vi "websocket main.vi"(8 "error in":errorcluster, 10 "upgrade data":T1, 11 "websocket handler in":refnum<class "websocket upgrade handler.lvclass">) -> (0 "error out":errorcluster)   [LabVIEW 2013, in "websocket upgrade handler.lvclass"]
uses:
  websocket upgrade handler.lvclass
  HTTP responder/http upgrade data.ctl
  HTTP server/http request.ctl
  HTTP server/http method.ctl
  HTTP headers/http header data.ctl
  websocket upgrade handler.lvclass/websocket upgrade handler.ctl
  user plugin/websocket user plugin.lvclass
  websocket core.lvlib
  HTTP server/Basic HTTP server.lvclass
  HTTP responder/http responder.lvclass
  HTTP headers/http headers.lvlib
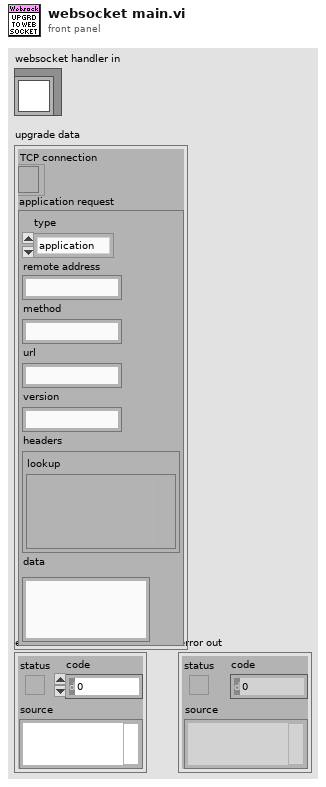
[diagram p1: front panel]
types:
  T1 = typedef "http responder.lvclass/http upgrade data.ctl" = cluster{"TCP connection":refnum<k5>, "application request":T2}
  T2 = typedef "Basic HTTP server.lvclass/http request.ctl" = cluster{"type":T3, "remote address":string, "method":string, "url":string, "version":string, "headers":T4, "data":string}
  T3 = typedef "Basic HTTP server.lvclass/http method.ctl" = enum16{"application", "error", "upgrade", "expect"}
  T4 = typedef "http headers.lvlib/http header data.ctl" = cluster{"lookup":variant}
  T5 = typedef "websocket core.lvlib/first byte header.ctl" = cluster{"fin":bool, "RSRV1":bool, "RSRV2":bool, "RSRV3":bool, "opcode":u8}
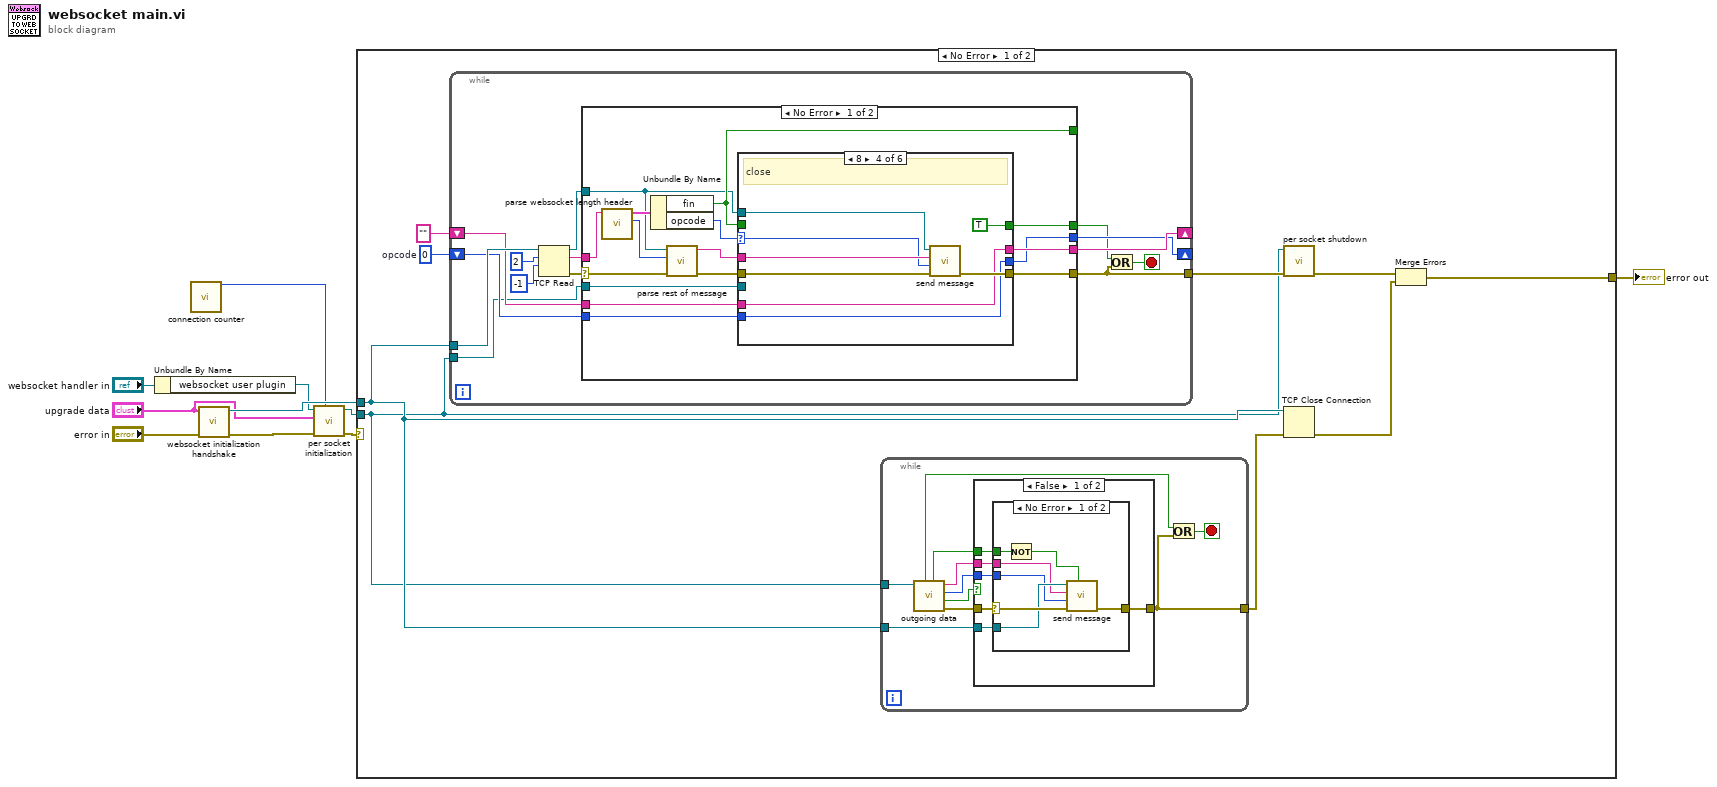
[diagram p0: block diagram]
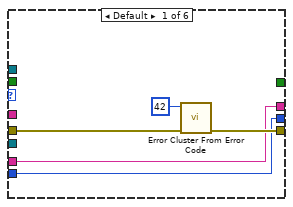
[diagram p4: hidden frame]
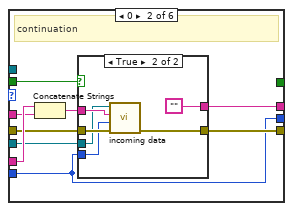
[diagram p5: hidden frame]
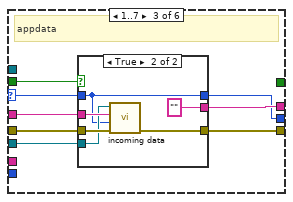
[diagram p7: hidden frame]
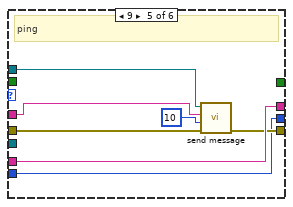
[diagram p9: hidden frame]
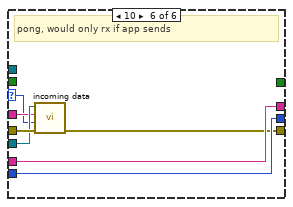
[diagram p10: hidden frame]
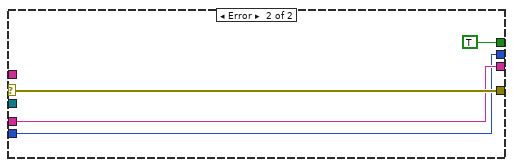
[diagram p11: hidden frame]
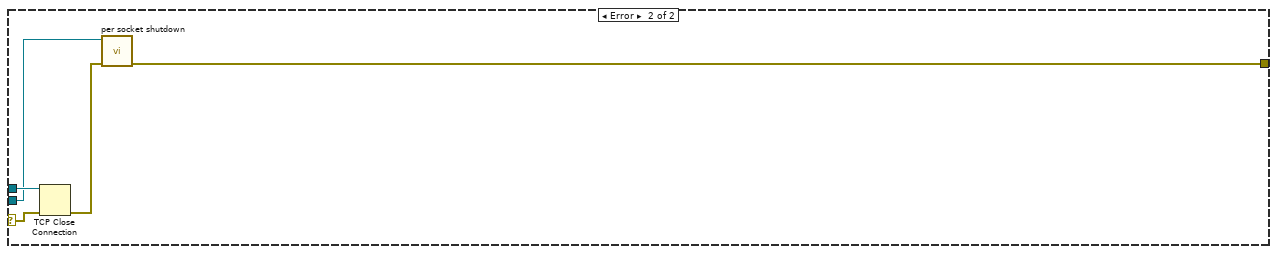
[diagram p12: hidden frame]
diagram:
  n1 = Unbundle By Name("websocket handler in") -> ("websocket user plugin"=w6:refnum<class "websocket user plugin.lvclass">)
  n2 = call "connection counter.vi"() -> ("id"=w1:i32)  [unwired: 11 in]
  n3 = call "websocket initialization handshake.vi"("error in"="error in", "upgrade data"="upgrade data") -> ("error out"=w4:errorcluster, "TCP Network Connection out"=w10:refnum<k5>)  [unwired: 8 in]
  n4 = call-dynamic "per socket initialization.vi"("id"=w1, "error in"=w4, "upgrade data"="upgrade data", "websocket user plugin in"=w6) -> ("error out"=w3:errorcluster, "websocket user plugin out"=w5:refnum<class "websocket user plugin.lvclass">)  [unwired: 6 in]
  n5 = case shown="No Error" w3 {
    selector: w3 -> [_ w143]
    tunnel: w10 -> [w12 w144]
    tunnel: [w14 w141] -> w8
    tunnel: w5 -> [w11 w140]
    frame No Error {
      w17 = u8 0  # opcode
      n6 = while {
        tunnel: w12 -> [w55]
        tunnel: [w52] -> w15
        shift-right: [w50] -> _
        shift-left: "" -> [w51]
        shift-right: [w48] -> _
        shift-left: w17 -> [w49]
        tunnel: w11 -> [w47]
        stop <- w46 stop-if-true
        n7 = TCP Read(connection ID=w55, bytes to read=2, 9:-1 ("timeout ms (25000)")) -> (connection ID out=w56:refnum<k5>, data out=w58:string, error out=w54:errorcluster)  [unwired: 2 in]
        n8 = case shown="No Error" w54 {
          selector: w54 -> [w74 w139]
          tunnel: w58 -> [w73 _]
          tunnel: w56 -> [w62 _]
          tunnel: [w70 w139] -> w52
          tunnel: w51 -> [w66 w138]
          tunnel: [w67 w138] -> w50
          tunnel: [w64 _] -> _
          tunnel: w49 -> [w59 w137]
          tunnel: [w60 w137] -> w48
          tunnel: w47 -> [w63 _]
          tunnel: [w61 TRUE] -> w45
          frame No Error {
            n9 = call "parse websocket length header.vi"("header string"=w73) -> ("mask(1)+length(7)"=w72:u8, "first byte"=w71:T5)  [unwired: 9 in]
            n10 = Unbundle By Name(w71) -> ("fin"=w64:bool, "opcode"=w68:u8)
            n11 = call "parse rest of message.vi"("error in"=w74, "mask(1)+length(7)"=w72, "TCP Network Connection in"=w62) -> ("error out"=w69:errorcluster, "unmasked data"=w65:string)  [unwired: 7 in]
            n12 = case shown="8" w68 {
              selector: w68 -> [_ _ w98 w116 _ w129]
              tunnel: [w78 w86 w104 w118 w123 w133] -> w70
              tunnel: w69 -> [w79 w85 w103 w119 w127 w132]
              tunnel: [w76 w82 w100 w115 w128 w135] -> w67
              tunnel: w66 -> [w76 w88 _ w115 w128 w135]
              tunnel: w65 -> [_ w87 w101 w121 w125 w130]
              tunnel: w64 -> [_ w84 w102 _ _ _]
              tunnel: w63 -> [_ w81 w99 _ _ w131]
              tunnel: w62 -> [_ _ _ w120 w124 _]
              tunnel: [_ _ _ TRUE _ _] -> w61
              tunnel: [w75 w80 w97 w114 w122 w134] -> w60
              tunnel: w59 -> [w75 w80 _ w114 w122 w134]
              frame Default {
                n13 = call <vilib>:"Error Cluster From Error Code.vi"("error in (no error)"=w79, "error code (0)"=42) -> ("error out"=w78:errorcluster)  [unwired: 7 in]
              }
              frame 0 {
                # "continuation"
                n14 = Concatenate Strings(w88, w87) -> (w83:string)
                n15 = case shown="True" w84 {
                  tunnel: [w90 w96] -> w86
                  tunnel: w85 -> [w90 w95]
                  tunnel: w83 -> [w89 w94]
                  tunnel: [w89 ""] -> w82
                  tunnel: w81 -> [_ w92]
                  tunnel: w80 -> [_ w91]
                  frame False {
                  }
                  frame True {
                    n16 = call-dynamic "incoming data.vi"("error in"=w95, "opcode"=w91, "data"=w94, "websocket user plugin in"=w92) -> ("error out"=w96:errorcluster)  [unwired: 7 in]
                  }
                }
              }
              frame 1..7 {
                # "appdata"
                n17 = case shown="True" w102 {
                  tunnel: [w107 w113] -> w104
                  tunnel: w103 -> [w107 w112]
                  tunnel: w101 -> [w106 w111]
                  tunnel: [w106 ""] -> w100
                  tunnel: w99 -> [_ w109]
                  tunnel: w98 -> [w105 w108]
                  tunnel: [w105 w108] -> w97
                  frame False {
                  }
                  frame True {
                    n18 = call-dynamic "incoming data.vi"("error in"=w112, "opcode"=w108, "data"=w111, "websocket user plugin in"=w109) -> ("error out"=w113:errorcluster)  [unwired: 7 in]
                  }
                }
              }
              frame 8 {
                # "close"
                n19 = call "send message.vi"("error in"=w119, "opcode"=w116, "data"=w121, "TCP Network Connection in"=w120) -> ("error out"=w118:errorcluster)  [unwired: 7 in]
              }
              frame 9 {
                # "ping"
                n20 = call "send message.vi"("error in"=w127, "opcode"=u8 10, "data"=w125, "TCP Network Connection in"=w124) -> ("error out"=w123:errorcluster)  [unwired: 7 in]
              }
              frame 10 {
                # "pong, would only rx if app sends"
                n21 = call-dynamic "incoming data.vi"("error in"=w132, "opcode"=w129, "data"=w130, "websocket user plugin in"=w131) -> ("error out"=w133:errorcluster)  [unwired: 7 in]
              }
            }
          }
          frame Error {
          }
        }
        n22 = Or(x=w45, y=w52) -> (x .or. y?=w46:bool)
      }
      n23 = while {
        tunnel: w12 -> [w29]
        tunnel: [w22] -> w16
        tunnel: w11 -> [w28]
        stop <- w21 stop-if-true
        n24 = call-dynamic "outgoing data.vi"("websocket user plugin in"=w28) -> ("error out"=w23:errorcluster, "timeout"=w24:bool, "opcode"=w25:u8, "data"=w26:string, "not last fragment (F)"=w27:bool, "kill connection"=w20:bool)  [unwired: 5 in]
        n25 = case shown="False" w24 {
          tunnel: w29 -> [w35 _]
          tunnel: [w34 w44] -> w22
          tunnel: w23 -> [w33 w44]
          tunnel: w27 -> [w32 _]
          tunnel: w26 -> [w31 _]
          tunnel: w25 -> [w30 _]
          frame False {
            n26 = case shown="No Error" w33 {
              selector: w33 -> [w41 w43]
              tunnel: [w42 w43] -> w34
              tunnel: w35 -> [w40 _]
              tunnel: w32 -> [w39 _]
              tunnel: w31 -> [w37 _]
              tunnel: w30 -> [w36 _]
              frame No Error {
                n27 = Not(x=w39) -> (.not. x?=w38:bool)
                n28 = call "send message.vi"("final fragment (T)"=w38, "error in"=w41, "opcode"=w36, "data"=w37, "TCP Network Connection in"=w40) -> ("error out"=w42:errorcluster)  [unwired: 6 in]
              }
              frame Error {
              }
            }
          }
          frame True {
          }
        }
        n29 = Or(x=w20, y=w22) -> (x .or. y?=w21:bool)
      }
      n30 = call-dynamic "per socket shutdown.vi"("error in (no error)"=w15, "websocket user plugin in"=w11) -> ("error out"=w19:errorcluster)  [unwired: 9 in]
      n31 = TCP Close Connection(connection ID=w12, error in (no error)=w16) -> (error out=w13:errorcluster)  [unwired: 1 in, 1 out]
      n32 = Merge Errors(w19, w13) -> (w14:errorcluster)
    }
    frame Error {
      n33 = TCP Close Connection(connection ID=w144, error in (no error)=w143) -> (error out=w142:errorcluster)  [unwired: 1 in, 1 out]
      n34 = call-dynamic "per socket shutdown.vi"("error in (no error)"=w142, "websocket user plugin in"=w140) -> ("error out"=w141:errorcluster)  [unwired: 9 in]
    }
  }
  "error out" <- w8
